vi "Tree_Select first or last item.vi"(7 "Select Item":enum16{"First", "Last"}(ring), 8 "error in (no error)":errorcluster, 11 "Tree Ref":refnum<vi>) -> (0 "error out":errorcluster, 3 "Tree Ref Out":refnum<vi>)   [LabVIEW 2023]
doc: "If last and down, go to first; if first and up, go to last."
panel:
  in  "Tree":string[](tree)
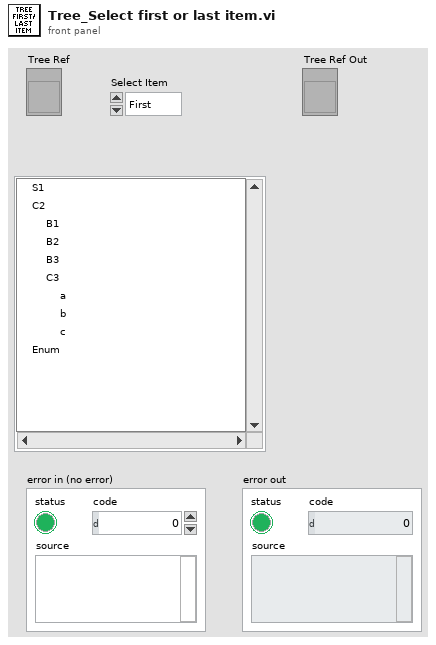
[diagram p1: front panel]
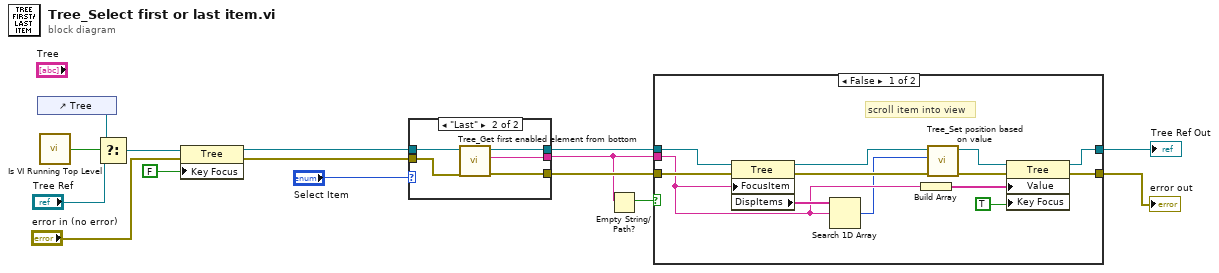
[diagram p0: block diagram]
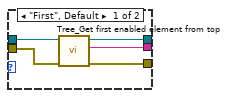
[diagram p3: hidden frame]
diagram:
  n1 = control-ref of="Tree"() -> (w14:refnum<vi>)
  n2 = call "Is VI Running Top Level.vi"() -> ("Top Level?"=w15:bool)  [unwired: 5 in]
  n3 = Select(t=w14, s=w15, f="Tree Ref") -> (s? t:f=w13:refnum<vi>)
  n4 = property class="Tree"(reference=w13, error in="error in (no error)", "Key Focus"=FALSE) -> (reference out=w8:refnum<vi>, error out=w5:errorcluster)
  n5 = case shown="\"Last\"" "Select Item" {
    tunnel: [w18 w23] -> w2
    tunnel: w8 -> [w20 w25]
    tunnel: [w19 w24] -> w7
    tunnel: w5 -> [w17 w22]
    tunnel: [w16 w21] -> w4
    frame "First", Default {
      n6 = call "Tree_Get first enabled element from top.vi"("error in (no error)"=w17, "Tree Control Ref"=w20) -> ("error out"=w16:errorcluster, "First Enabled Element"=w18:string, "Tree Control Ref Out"=w19:refnum<vi>)  [unwired: 7 in]
    }
    frame "Last" {
      n7 = call "Tree_Get first enabled element from bottom.vi"("error in (no error)"=w22, "TreeControl Ref"=w25) -> ("error out"=w21:errorcluster, "First Element Tag"=w23:string, "Tree Control Ref Out"=w24:refnum<vi>)  [unwired: 7 in]
    }
  }
  n8 = Empty String/Path?(string/path=w2) -> (empty?=w1:bool)
  n9 = case shown="False" w1 {
    tunnel: [w36 w40] -> w9
    tunnel: w7 -> [w35 w40]
    tunnel: w4 -> [w33 w39]
    tunnel: w2 -> [w29 _]
    tunnel: [w26 w39] -> w3
    frame False {
      # "scroll item into view"
      n10 = property class="Tree"(reference=w35, error in=w33, "FocusItem"=w29) -> (reference out=w34:refnum<vi>, error out=w32:errorcluster, "DispItems"=w30:string[])
      n11 = Search 1D Array(1D array=w30, element=w29) -> (index of element=w28:i32)  [unwired: 1 in]
      n12 = Build Array(w29) -> (w27:string[])
      n13 = call "Tree_Set position based on value.vi"("error in (no error)"=w32, "Selected Row"=w28, "Tree Ref"=w34) -> ("error out"=w31:errorcluster, "Tree Ref"=w37:refnum<vi>)  [unwired: 7 in]
      n14 = property class="Tree"(reference=w37, error in=w31, "Value"=w27, "Key Focus"=TRUE) -> (reference out=w36:refnum<vi>, error out=w26:errorcluster)
    }
    frame True {
    }
  }
  "Tree Ref Out" <- w9
  "error out" <- w3
